vi "Periodic Tasks.vi"(8 "error in":errorcluster) -> ()   [LabVIEW 2015]
doc: "This VI runs in parallel to other tasks. It can contain as many user-defined periodic loops as you need. These can carry out PID or other sorts of timed response."
uses:
  Robot Global Data.vi
  <vilib>/Rock Robotics/WPI/Ultrasonic/WPI_SonarMB1010DigitalRefNum Registry Get.vi
  <vilib>/Rock Robotics/WPI/Ultrasonic/WPI_SonarMB1010DigitalGetRange.vi
  <vilib>/addons/control/pid/pid.llb/PID (DBL).vi
  navx-mxp/labview/navX Library v2/navX Library v2.lvlib
  <vilib>/addons/control/pid/NI_PID_pid.lvlib
panel:
  in  "Amperage setpoint":dbl=4.5 format="%#_13g"
  out "current (A)":dbl
  out "Pitch":dbl
  in  "PID gains 2":T1={"proportional gain (Kc)"=6.0, "integral time (Ti, min)"=0.0, "derivative time (Td, min)"=0.0}
  in  "Level 1":dbl=0.106 format="%#_13g"
  in  "Level 2":dbl=0.2 format="%#_13g"
  in  "Level 3":dbl=0.845 format="%#_13g"
  out "Motor Output":dbl(graph)
  in  "PID gains":T1={"proportional gain (Kc)"=7.0, "integral time (Ti, min)"=0.0, "derivative time (Td, min)"=0.00045}
  out "Distance":dbl
  out "Potentiometer":dbl
  out "Beam Brake Tripped?":bool
  out "Yaw":dbl
  out "Roll":dbl
  in  "Command limit":dbl=0.25
  in  "Yaw Reset":bool
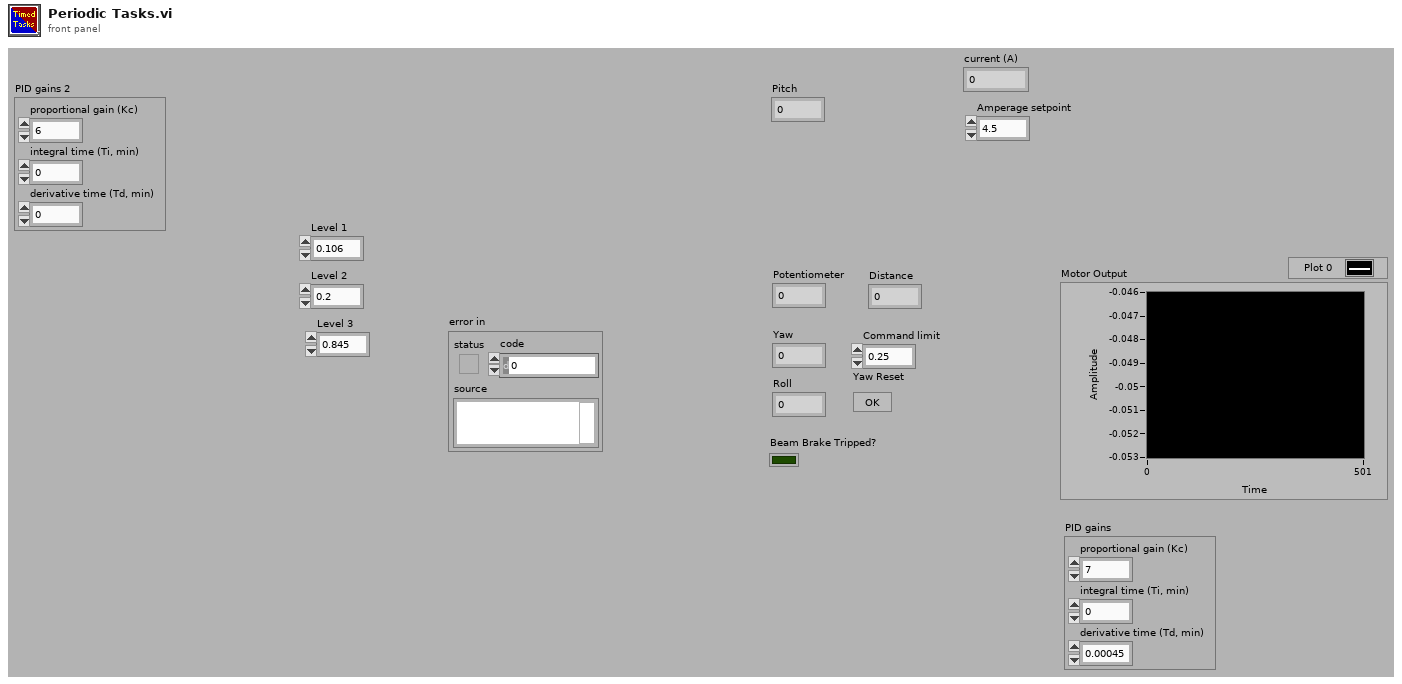
[diagram p1: front panel]
types:
  T1 = cluster{"proportional gain (Kc)":dbl, "integral time (Ti, min)":dbl, "derivative time (Td, min)":dbl}
  T2 = typedef "WPI_MotorControlDeviceRef.ctl" = cluster{"DeviceStatus":errorcluster, "Type":T3, "PWM":cluster{"PWM Channel":T4, "DeadBand":T5}, "CAN":cluster{"Device Number":u8, "Control Mode":T6, "Semaphore":T7, "Max Vout":dbl, "TalonSRX Control Mode":T8}, "Invert":bool}
  T3 = typedef "WPI_MotorControlType.ctl" = enum16{"PWM", "CAN", "CANTalonSRX"}
  T4 = typedef "FPGA_DIOPWMChannel.ctl" = enum8{"PWM 0", "PWM 1", "PWM 2", "PWM 3", "PWM 4", "PWM 5", "PWM 6", "PWM 7", "PWM 8", "PWM 9", "PWM MXP 0", "PWM MXP 1", "PWM MXP 2", "PWM MXP 3", "PWM MXP 4", "PWM MXP 5", "PWM MXP 6", "PWM MXP 7", "PWM MXP 8", "PWM MXP 9", "Invalid"}
  T5 = typedef "WPI_PWMDeadband.ctl" = cluster{"Name":string, "maxPositivePwm":i32, "minPositivePwm":i32, "centerPwm":i32, "maxNegativePwm":i32, "minNegativePwm":i32, "angularRange":u16}
  T6 = typedef "WPI_CANJaguar_ControlMode.ctl" = enum8{"Percent VBus", "Current", "Speed", "Position", "Voltage"}
  T7 = typedef "Semaphore RefNum" = refnum<k1>
  T8 = typedef "WPI_CANTalonSRX_APIControlMode.ctl" = enum8{"Percent VBus", "Speed", "Position", "Slave", "Unchanged / Invalid", "Voltage Compensation", "Current", "Motion Profile"}
  T9 = typedef "WPI_PotentiometerDevRef.ctl" = cluster{"DevStatus":errorcluster, "Analog Channel":T10, "Invert Output":bool}
  T10 = typedef "FPGA_AIChannel.ctl" = enum8{"AI 0", "AI 1", "AI 2", "AI 3", "AI MXP 0", "AI MXP 1", "AI MXP 2", "AI MXP 3", "Invalid"}
  T11 = typedef "WPI_DigitalInputDevRef.ctl" = cluster{"DevStatus":errorcluster, "DIO Channel":T12}
  T12 = typedef "FPGA_DIOChannel.ctl" = enum8{"DIO 0", "DIO 1", "DIO 2", "DIO 3", "DIO 4", "DIO 5", "DIO 6", "DIO 7", "DIO 8", "DIO 9", "DIO MXP 0", "DIO MXP 1", "DIO MXP 2", "DIO MXP 3", "DIO MXP 4", "DIO MXP 5", "DIO MXP 6", "DIO MXP 7", "DIO MXP 8", "DIO MXP 9", "DIO MXP 10", "DIO MXP 11", "DIO MXP 12", "DIO MXP 13", "DIO MXP 14", "DIO MXP 15", "Invalid"}
  T13 = typedef "WPI_SonarMB1010DigitalDeviceRef.ctl" = cluster{"CounterDevRef":T14, "Scaling factor (s/in)":dbl}
  T14 = typedef "WPI_CounterDevRef.ctl" = cluster{"DevStatus":errorcluster, "CntIndex":T15}
  T15 = typedef "FPGA_CounterCtrSystemIndex.ctl" = enum8{"Ctr 0", "Ctr 1", "Ctr 2", "Ctr 3", "Ctr 4", "Ctr 5", "Ctr 6", "Ctr 7", "Invalid"}
  T16 = typedef "navX Library v2.lvlib/Z900_navX_DeviceTypeDef.ctl" = cluster{"Interface":cluster{"Protocol":T17, "Update Rate (4Hz-60Hz)":u8, "navX Open TypeDef":variant}, "Notify Packet":refnum<notifier>, "Loop VI Refnum":refnum<vi>, "Ready to Close Occurrence Refnum":refnum<k4>}
  T17 = typedef "navX Library v2.lvlib/Z900_navX_ProtocolTypeDef.ctl" = enum16{"SERIAL", "I2C", "SPI"}
  T18 = cluster{"Yaw":dbl, "Roll":dbl, "Pitch":dbl, "Heading":dbl, "Fused Heading":dbl}
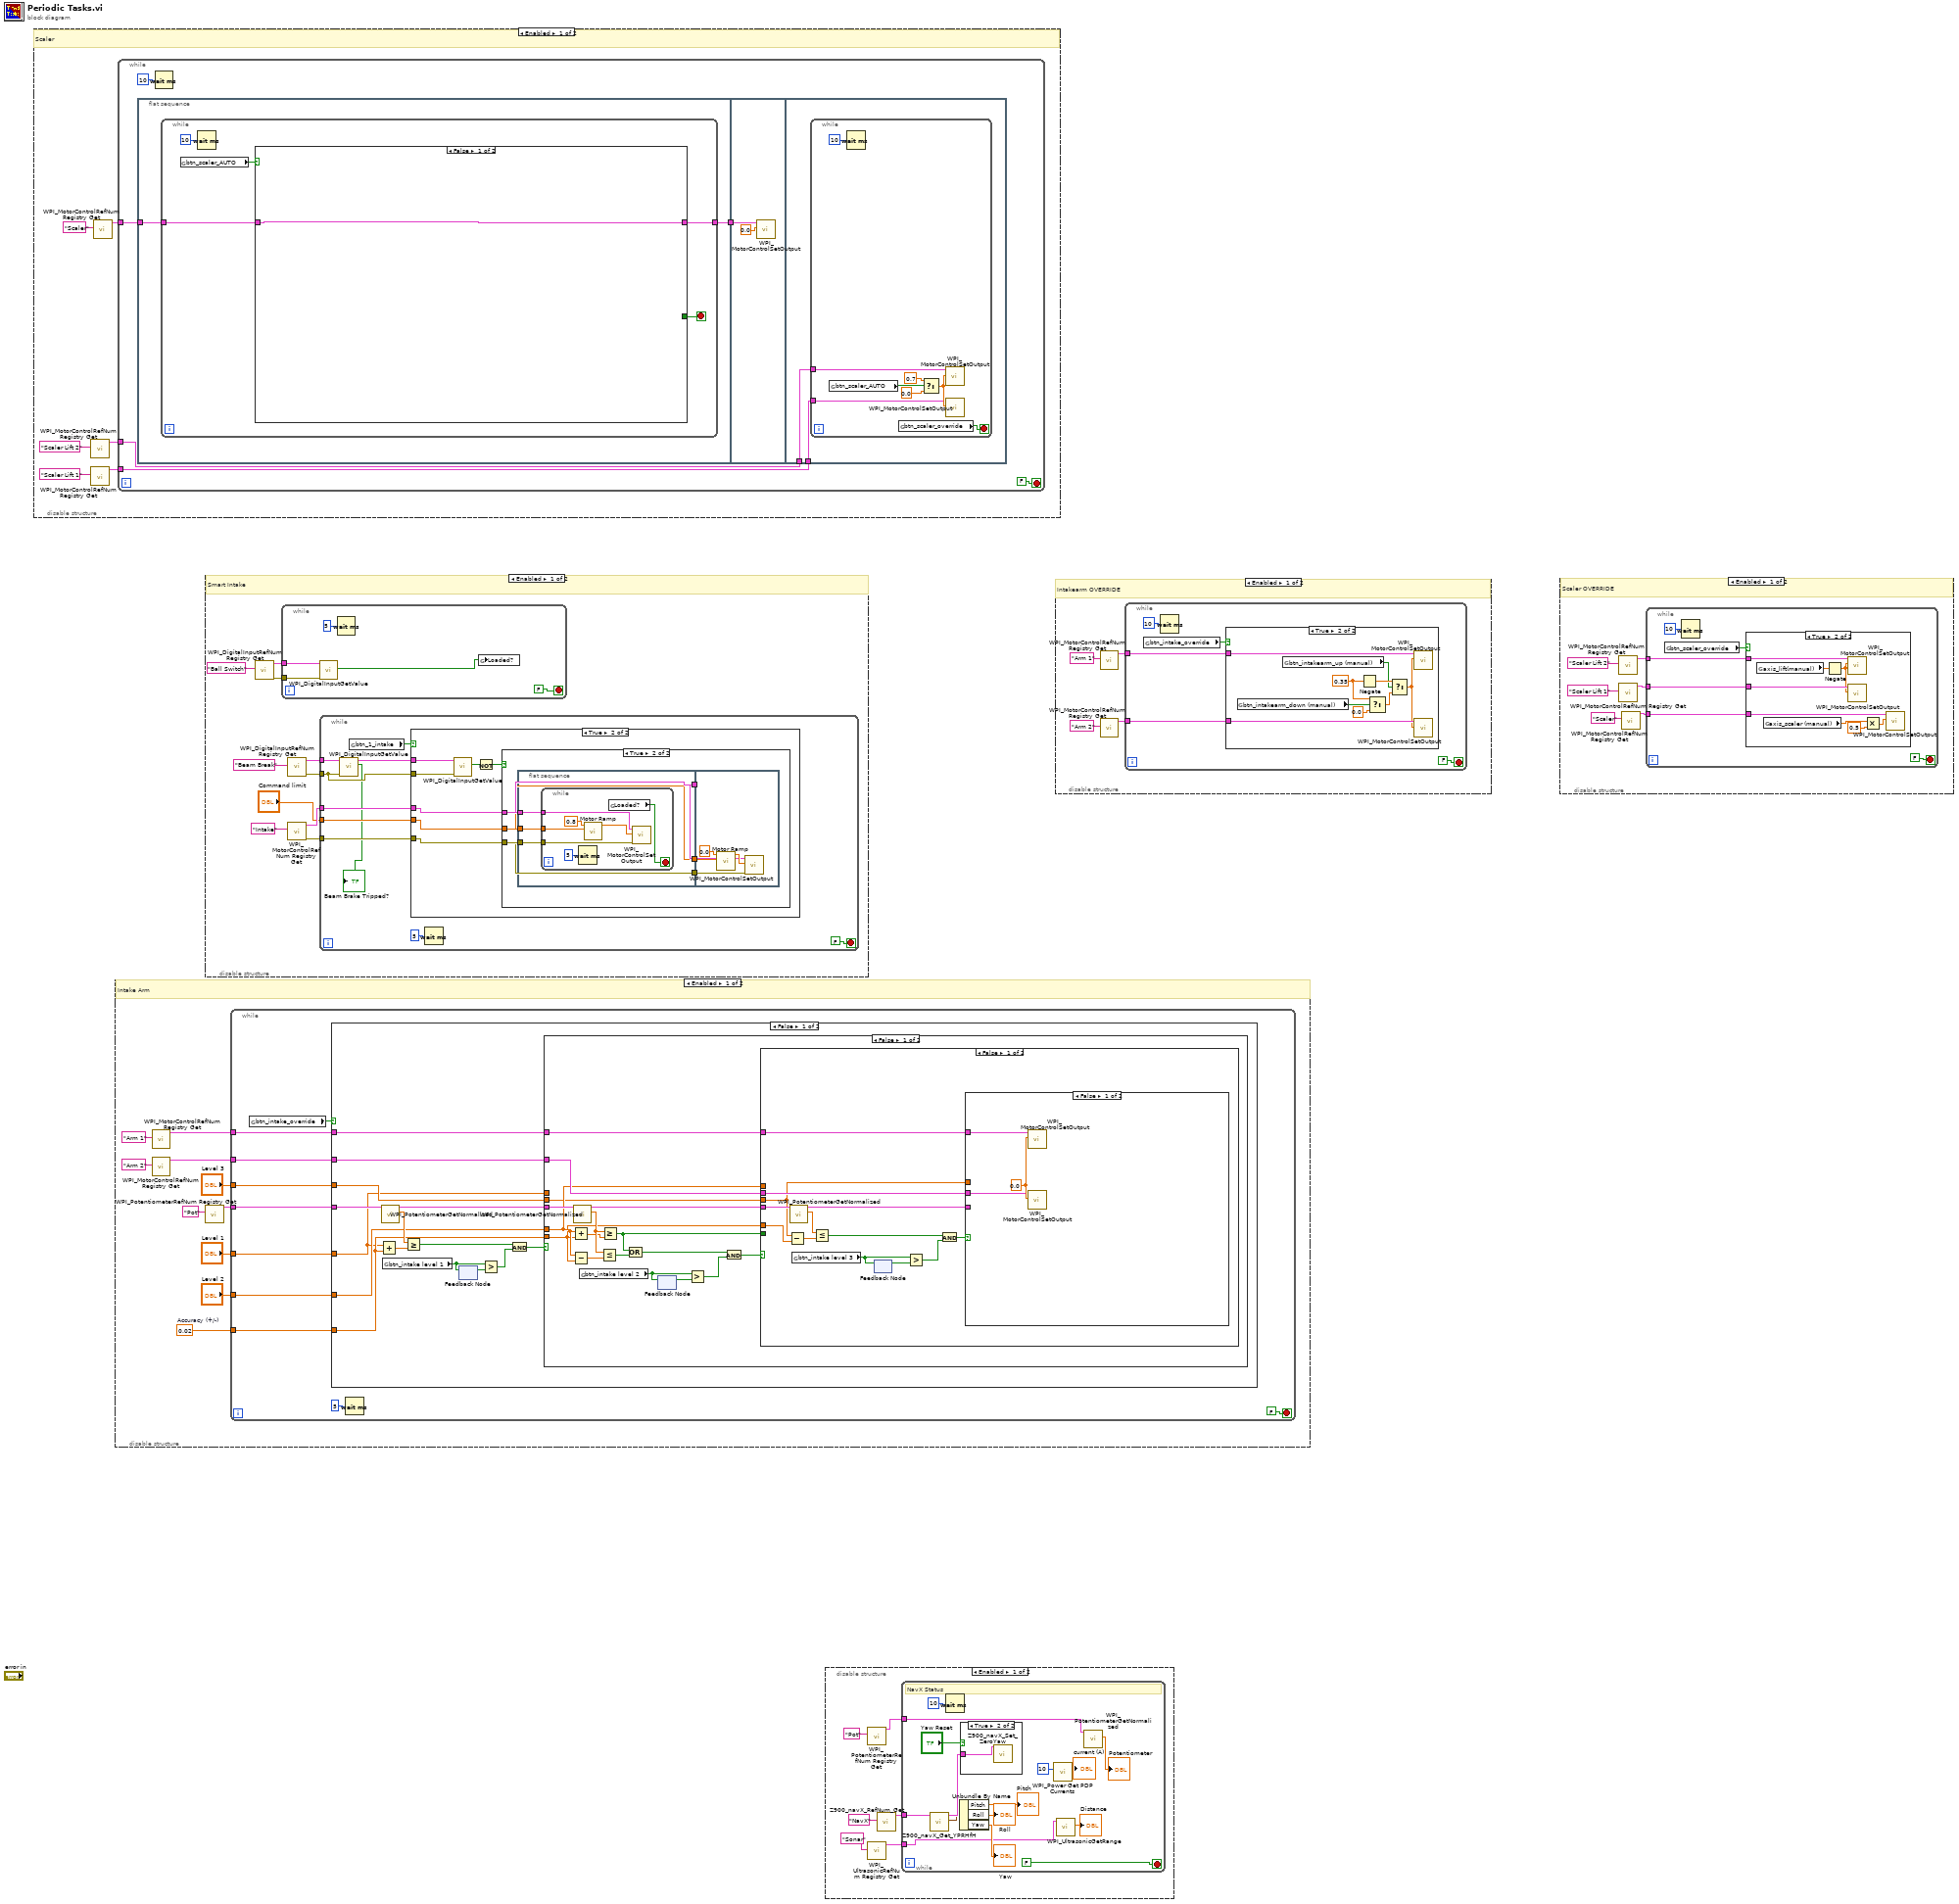
[diagram p0: block diagram]
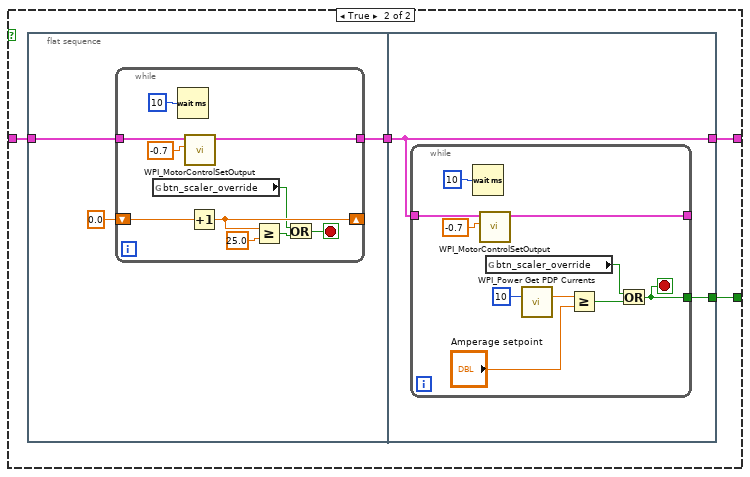
[diagram p2: hidden frame]
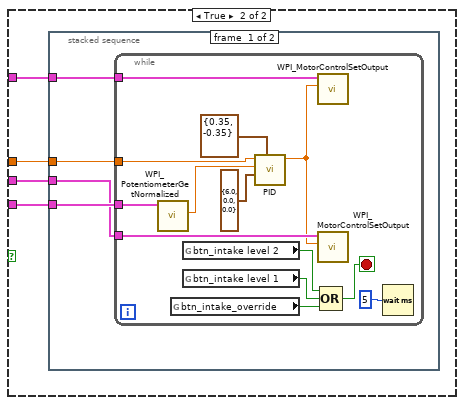
[diagram p8: hidden frame]
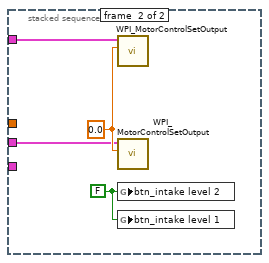
[diagram p9: hidden frame]
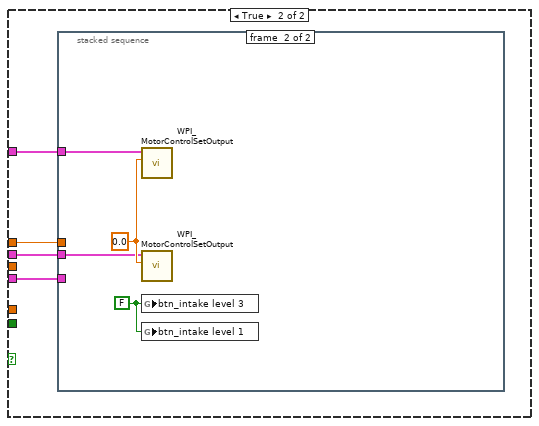
[diagram p10: hidden frame]
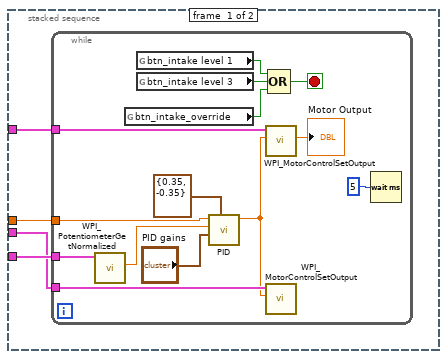
[diagram p11: hidden frame]
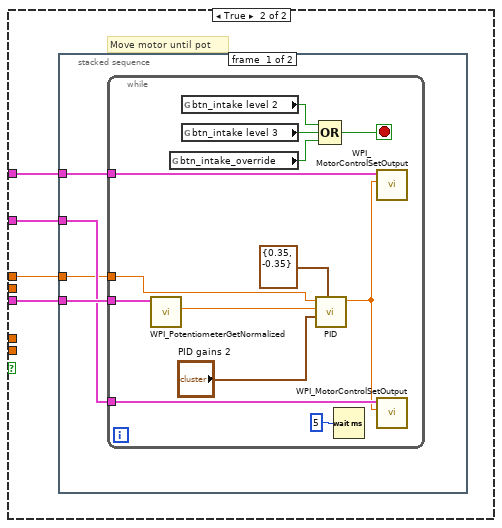
[diagram p12: hidden frame]
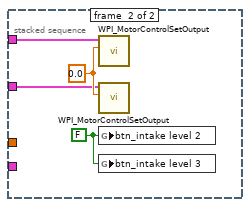
[diagram p13: hidden frame]
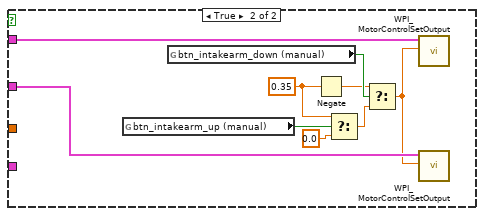
[diagram p14: hidden frame]
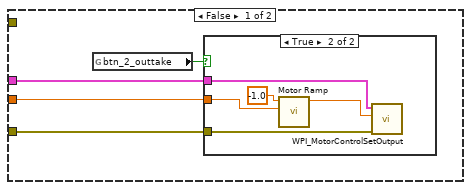
[diagram p18: hidden frame]
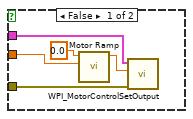
[diagram p19: hidden frame]
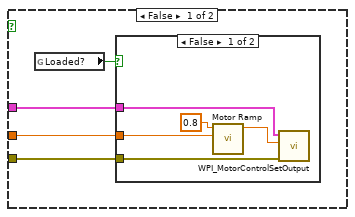
[diagram p20: hidden frame]
diagram:
  n1 = disable-structure shown="Enabled" {
    frame Enabled {
      # "Scaler"
      n2 = call <vilib>:"WPI_MotorControlRefNum Registry Get.vi"("refnum name"="Scaler Lift 2") -> ("MotorControlDevRef"=w2:T2)  [unwired: 9 in, 1 out]
      n3 = call <vilib>:"WPI_MotorControlRefNum Registry Get.vi"("refnum name"="Scaler Lift 1") -> ("MotorControlDevRef"=w1:T2)  [unwired: 9 in, 1 out]
      n4 = call <vilib>:"WPI_MotorControlRefNum Registry Get.vi"("refnum name"="Scaler") -> ("MotorControlDevRef"=w3:T2)  [unwired: 9 in, 1 out]
      n5 = while {
        tunnel: w3 -> [w10]
        tunnel: w2 -> [w8]
        tunnel: w1 -> [w7]
        stop <- FALSE stop-if-true
        n6 = flat-sequence {
          tunnel: w10 -> [w14]
          tunnel: [w13] -> w9
          tunnel: w9 -> [w51]
          tunnel: w8 -> [w53]
          tunnel: w7 -> [w52]
          frame #0 {
            n7 = while {
              tunnel: w14 -> [w18]
              tunnel: [w17] -> w13
              stop <- w16 stop-if-true
              n8 = global read "Robot Global Data.vi" "btn_scaler_AUTO"() -> (w19:bool)
              n9 = Wait (ms)(milliseconds to wait=u32 10) -> ()  [unwired: 1 out]
              n10 = case shown="False" w19 {
                tunnel: w18 -> [w20 w24]
                tunnel: [w20 w23] -> w17
                tunnel: [_ w21] -> w16
                frame False {
                }
                frame True {
                  n11 = flat-sequence {
                    tunnel: w24 -> [w27]
                    tunnel: [w26] -> w22
                    tunnel: [w39] -> w23
                    tunnel: w22 -> [w39]
                    tunnel: [w38] -> w21
                    frame #0 {
                      n12 = while {
                        tunnel: w27 -> [w37]
                        tunnel: [w36] -> w26
                        shift-right: [w31] -> _
                        shift-left: 0.0 -> [w33]
                        stop <- w30 stop-if-true
                        n13 = global read "Robot Global Data.vi" "btn_scaler_override"() -> (w29:bool)
                        n14 = Wait (ms)(milliseconds to wait=u32 10) -> ()  [unwired: 1 out]
                        n15 = call <vilib>:"WPI_MotorControlSetOutput.vi"("Output"=-0.7, "MotorControlDevRef"=w37) -> ("MotorControlDevRef"=w36:T2)  [unwired: 7 in, 2 out]
                        n16 = Increment(x=w33) -> (x+1=w31:dbl)
                        n17 = Greater Or Equal?(x=w31, y=25.0) -> (x >= y?=w28:bool)
                        n18 = Or(x=w29, y=w28) -> (x .or. y?=w30:bool)
                      }
                    }
                    frame #1 {
                      n19 = while {
                        tunnel: [w49] -> _
                        tunnel: w39 -> [w45]
                        tunnel: [w40] -> w38
                        stop <- w40 stop-if-true
                        n20 = Wait (ms)(milliseconds to wait=u32 10) -> ()  [unwired: 1 out]
                        n21 = call <vilib>:"WPI_MotorControlSetOutput.vi"("Output"=-0.7, "MotorControlDevRef"=w45) -> ("MotorControlDevRef"=w49:T2)  [unwired: 7 in, 2 out]
                        n22 = global read "Robot Global Data.vi" "btn_scaler_override"() -> (w46:bool)
                        n23 = call <vilib>:"WPI_Power Get PDP Currents.vi"("PDP Channel"=10) -> ("current (A)"=w43:dbl)  [unwired: 12 in, 2 out]
                        n24 = Greater Or Equal?(x=w43, y="Amperage setpoint") -> (x >= y?=w42:bool)
                        n25 = Or(x=w46, y=w42) -> (x .or. y?=w40:bool)
                      }
                    }
                  }
                }
              }
            }
          }
          frame #1 {
            n26 = call <vilib>:"WPI_MotorControlSetOutput.vi"("Output"=0.0, "MotorControlDevRef"=w51) -> ()  [unwired: 7 in, 3 out]
          }
          frame #2 {
            n27 = while {
              tunnel: w53 -> [w55]
              tunnel: w52 -> [w54]
              stop <- w60 stop-if-true
              n28 = global read "Robot Global Data.vi" "btn_scaler_AUTO"() -> (w59:bool)
              n29 = Wait (ms)(milliseconds to wait=u32 10) -> ()  [unwired: 1 out]
              n30 = global read "Robot Global Data.vi" "btn_scaler_override"() -> (w60:bool)
              n31 = Select(t=0.7, s=w59, f=0.0) -> (s? t:f=w56:dbl)
              n32 = call <vilib>:"WPI_MotorControlSetOutput.vi"("Output"=w56, "MotorControlDevRef"=w55) -> ()  [unwired: 7 in, 3 out]
              n33 = call <vilib>:"WPI_MotorControlSetOutput.vi"("Output"=w56, "MotorControlDevRef"=w54) -> ()  [unwired: 7 in, 3 out]
            }
          }
        }
        n34 = Wait (ms)(milliseconds to wait=u32 10) -> ()  [unwired: 1 out]
      }
    }
    frame Disabled {
    }
  }
  n35 = disable-structure shown="Enabled" {
    frame Enabled {
      w65 = 0.02  # Accuracy (+/-)
      # "Intake Arm"
      n36 = call <vilib>:"WPI_MotorControlRefNum Registry Get.vi"("refnum name"="Arm 1") -> ("MotorControlDevRef"=w67:T2)  [unwired: 9 in, 1 out]
      n37 = call <vilib>:"WPI_MotorControlRefNum Registry Get.vi"("refnum name"="Arm 2") -> ("MotorControlDevRef"=w66:T2)  [unwired: 9 in, 1 out]
      n38 = call <vilib>:"WPI_PotentiometerRefNum Registry Get.vi"("refnum name"="Pot") -> ("PotDevRef"=w68:T9)  [unwired: 9 in, 1 out]
      n39 = while {
        tunnel: w68 -> [w80]
        tunnel: w67 -> [w79]
        tunnel: w66 -> [w78]
        tunnel: w65 -> [w76]
        tunnel: "Level 3" -> [w75]
        tunnel: "Level 2" -> [w74]
        tunnel: "Level 1" -> [w73]
        stop <- FALSE stop-if-true
        n40 = global read "Robot Global Data.vi" "btn_intake_override"() -> (w72:bool)
        n41 = case shown="False" w72 {
          tunnel: w80 -> [w91 _]
          tunnel: w79 -> [w89 w214]
          tunnel: w78 -> [w88 w213]
          tunnel: w76 -> [w85 _]
          tunnel: w75 -> [w84 _]
          tunnel: w74 -> [w83 _]
          tunnel: w73 -> [w82 _]
          frame False {
            n42 = Add(x=w82, y=w85) -> (x+y=w86:dbl)
            n43 = call <vilib>:"WPI_PotentiometerGetNormalized.vi"("PotDevRef"=w91) -> ("Normalized Value"=w87:dbl, "PotDevRef"=w90:T9)  [unwired: 8 in, 1 out]
            n44 = global read "Robot Global Data.vi" "btn_intake level 1"() -> (w92:bool)
            n45 = Greater Or Equal?(x=w87, y=w86) -> (x >= y?=w95:bool)
            n46 = feedback #1() -> (w93:bool)  [unwired: 1 in]
            n47 = feedback-in #1(w92) -> ()
            n48 = Greater?(x=w92, y=w93) -> (0:w94:bool)
            n49 = And(x=w95, y=w94) -> (x .and. y?=w96:bool)
            n50 = case shown="False" w96 {
              tunnel: w90 -> [w106 w184]
              tunnel: w89 -> [w103 w183]
              tunnel: w88 -> [w102 w182]
              tunnel: w83 -> [w99 _]
              tunnel: w85 -> [w98 _]
              tunnel: w84 -> [w97 _]
              tunnel: w82 -> [_ w181]
              frame False {
                n51 = Add(x=w99, y=w98) -> (x+y=w101:dbl)
                n52 = Subtract(x=w99, y=w98) -> (x-y=w100:dbl)
                n53 = call <vilib>:"WPI_PotentiometerGetNormalized.vi"("PotDevRef"=w106) -> ("Normalized Value"=w107:dbl, "PotDevRef"=w105:T9)  [unwired: 8 in, 1 out]
                n54 = global read "Robot Global Data.vi" "btn_intake level 2"() -> (w108:bool)
                n55 = Less Or Equal?(x=w107, y=w100) -> (x <= y?=w112:bool)
                n56 = Greater Or Equal?(x=w107, y=w101) -> (x >= y?=w104:bool)
                n57 = Or(x=w104, y=w112) -> (x .or. y?=w110:bool)
                n58 = feedback #2() -> (w113:bool)  [unwired: 1 in]
                n59 = feedback-in #2(w108) -> ()
                n60 = Greater?(x=w108, y=w113) -> (0:w111:bool)
                n61 = And(x=w110, y=w111) -> (x .and. y?=w109:bool)
                n62 = case shown="False" w109 {
                  tunnel: w105 -> [w120 w158]
                  tunnel: w104 -> [_ _]
                  tunnel: w103 -> [w117 w157]
                  tunnel: w102 -> [w118 w156]
                  tunnel: w99 -> [_ w155]
                  tunnel: w98 -> [w115 _]
                  tunnel: w97 -> [w114 _]
                  frame False {
                    n63 = Subtract(x=w114, y=w115) -> (x-y=w116:dbl)
                    n64 = call <vilib>:"WPI_PotentiometerGetNormalized.vi"("PotDevRef"=w120) -> ("Normalized Value"=w121:dbl, "PotDevRef"=w119:T9)  [unwired: 8 in, 1 out]
                    n65 = global read "Robot Global Data.vi" "btn_intake level 3"() -> (w122:bool)
                    n66 = Less Or Equal?(x=w121, y=w116) -> (x <= y?=w124:bool)
                    n67 = feedback #3() -> (w126:bool)  [unwired: 1 in]
                    n68 = feedback-in #3(w122) -> ()
                    n69 = Greater?(x=w122, y=w126) -> (0:w125:bool)
                    n70 = And(x=w124, y=w125) -> (x .and. y?=w123:bool)
                    n71 = case shown="False" w123 {
                      tunnel: w119 -> [_ w133]
                      tunnel: w118 -> [w127 w132]
                      tunnel: w117 -> [w128 w131]
                      tunnel: w114 -> [_ w130]
                      frame False {
                        w129 = 0.0 ("Output")
                        n72 = call <vilib>:"WPI_MotorControlSetOutput.vi"("Output"=w129, "MotorControlDevRef"=w128) -> ()  [unwired: 7 in, 3 out]
                        n73 = call <vilib>:"WPI_MotorControlSetOutput.vi"("Output"=w129, "MotorControlDevRef"=w127) -> ()  [unwired: 7 in, 3 out]
                      }
                      frame True {
                        n74 = stacked-sequence {
                          tunnel: w133 -> [w137 _]
                          tunnel: w132 -> [w136 w153]
                          tunnel: w131 -> [w135 w152]
                          tunnel: w130 -> [w134 _]
                          frame #0 {
                            n75 = while {
                              tunnel: w137 -> [w149]
                              tunnel: w136 -> [w148]
                              tunnel: w135 -> [w147]
                              tunnel: w134 -> [w139]
                              stop <- w140 stop-if-true
                              n76 = call <vilib>:"WPI_PotentiometerGetNormalized.vi"("PotDevRef"=w149) -> ("Normalized Value"=w143:dbl)  [unwired: 8 in, 2 out]
                              n77 = global read "Robot Global Data.vi" "btn_intake_override"() -> (w138:bool)
                              n78 = global read "Robot Global Data.vi" "btn_intake level 2"() -> (w142:bool)
                              n79 = global read "Robot Global Data.vi" "btn_intake level 1"() -> (w141:bool)
                              n80 = call-poly <vilib>:"PID.vi"("output range"=cluster{"output high":dbl, "output low":dbl} {"output high"=0.35, "output low"=-0.35}, "PID gains"=T1 {"proportional gain (Kc)"=6.0, "integral time (Ti, min)"=0.0, "derivative time (Td, min)"=0.0}, "process variable"=w143, "setpoint"=w139) -> ("output"=w146:dbl)  [unwired: 6 in, 1 out]
                              n81 = call <vilib>:"WPI_MotorControlSetOutput.vi"("Output"=w146, "MotorControlDevRef"=w147) -> ()  [unwired: 7 in, 3 out]
                              n82 = call <vilib>:"WPI_MotorControlSetOutput.vi"("Output"=w146, "MotorControlDevRef"=w148) -> ()  [unwired: 7 in, 3 out]
                              n83 = Compound Arithmetic op=OR(w142, w141, w138) -> (w140:bool)
                              n84 = Wait (ms)(milliseconds to wait=u32 5) -> ()  [unwired: 1 out]
                            }
                          }
                          frame #1 {
                            w151 = FALSE ("btn_intake level 2")
                            w154 = 0.0 ("Output")
                            n85 = call <vilib>:"WPI_MotorControlSetOutput.vi"("Output"=w154, "MotorControlDevRef"=w152) -> ()  [unwired: 7 in, 3 out]
                            n86 = call <vilib>:"WPI_MotorControlSetOutput.vi"("Output"=w154, "MotorControlDevRef"=w153) -> ()  [unwired: 7 in, 3 out]
                            n87 = global write "Robot Global Data.vi" "btn_intake level 2"(w151) -> ()
                            n88 = global write "Robot Global Data.vi" "btn_intake level 1"(w151) -> ()
                          }
                        }
                      }
                    }
                  }
                  frame True {
                    n89 = stacked-sequence {
                      tunnel: w158 -> [w162 _]
                      tunnel: w157 -> [w161 w178]
                      tunnel: w156 -> [w160 w179]
                      tunnel: w155 -> [w159 _]
                      frame #0 {
                        n90 = while {
                          tunnel: w162 -> [w175]
                          tunnel: w161 -> [w174]
                          tunnel: w160 -> [w173]
                          tunnel: w159 -> [w165]
                          stop <- w166 stop-if-true
                          n91 = call <vilib>:"WPI_PotentiometerGetNormalized.vi"("PotDevRef"=w175) -> ("Normalized Value"=w169:dbl)  [unwired: 8 in, 2 out]
                          n92 = global read "Robot Global Data.vi" "btn_intake_override"() -> (w163:bool)
                          n93 = global read "Robot Global Data.vi" "btn_intake level 1"() -> (w168:bool)
                          n94 = global read "Robot Global Data.vi" "btn_intake level 3"() -> (w167:bool)
                          n95 = call-poly <vilib>:"PID.vi"("output range"=cluster{"output high":dbl, "output low":dbl} {"output high"=0.35, "output low"=-0.35}, "PID gains"="PID gains", "process variable"=w169, "setpoint"=w165) -> ("output"=w170:dbl)  [unwired: 6 in, 1 out]
                          n96 = call <vilib>:"WPI_MotorControlSetOutput.vi"("Output"=w170, "MotorControlDevRef"=w174) -> ("Motor Output"=→"Motor Output":dbl)  [unwired: 7 in, 2 out]
                          n97 = call <vilib>:"WPI_MotorControlSetOutput.vi"("Output"=w170, "MotorControlDevRef"=w173) -> ()  [unwired: 7 in, 3 out]
                          n98 = Compound Arithmetic op=OR(w168, w167, w163) -> (w166:bool)
                          n99 = Wait (ms)(milliseconds to wait=u32 5) -> ()  [unwired: 1 out]
                        }
                      }
                      frame #1 {
                        w177 = FALSE ("btn_intake level 2")
                        w180 = 0.0 ("Output")
                        n100 = call <vilib>:"WPI_MotorControlSetOutput.vi"("Output"=w180, "MotorControlDevRef"=w178) -> ()  [unwired: 7 in, 3 out]
                        n101 = call <vilib>:"WPI_MotorControlSetOutput.vi"("Output"=w180, "MotorControlDevRef"=w179) -> ()  [unwired: 7 in, 3 out]
                        n102 = global write "Robot Global Data.vi" "btn_intake level 3"(w177) -> ()
                        n103 = global write "Robot Global Data.vi" "btn_intake level 1"(w177) -> ()
                      }
                    }
                  }
                }
              }
              frame True {
                # "Move motor until pot"
                n104 = stacked-sequence {
                  tunnel: w184 -> [w188 _]
                  tunnel: w183 -> [w187 w204]
                  tunnel: w182 -> [w186 w203]
                  tunnel: w181 -> [w185 _]
                  frame #0 {
                    n105 = while {
                      tunnel: w188 -> [w200]
                      tunnel: w187 -> [w199]
                      tunnel: w186 -> [w198]
                      tunnel: w185 -> [w190]
                      stop <- w191 stop-if-true
                      n106 = call <vilib>:"WPI_PotentiometerGetNormalized.vi"("PotDevRef"=w200) -> ("Normalized Value"=w192:dbl)  [unwired: 8 in, 2 out]
                      n107 = global read "Robot Global Data.vi" "btn_intake_override"() -> (w189:bool)
                      n108 = global read "Robot Global Data.vi" "btn_intake level 2"() -> (w195:bool)
                      n109 = global read "Robot Global Data.vi" "btn_intake level 3"() -> (w194:bool)
                      n110 = call-poly <vilib>:"PID.vi"("output range"=cluster{"output high":dbl, "output low":dbl} {"output high"=0.35, "output low"=-0.35}, "PID gains"="PID gains 2", "process variable"=w192, "setpoint"=w190) -> ("output"=w193:dbl)  [unwired: 6 in, 1 out]
                      n111 = Compound Arithmetic op=OR(w195, w194, w189) -> (w191:bool)
                      n112 = Wait (ms)(milliseconds to wait=u32 5) -> ()  [unwired: 1 out]
                      n113 = call <vilib>:"WPI_MotorControlSetOutput.vi"("Output"=w193, "MotorControlDevRef"=w199) -> ()  [unwired: 7 in, 3 out]
                      n114 = call <vilib>:"WPI_MotorControlSetOutput.vi"("Output"=w193, "MotorControlDevRef"=w198) -> ()  [unwired: 7 in, 3 out]
                    }
                  }
                  frame #1 {
                    w202 = FALSE ("btn_intake level 2")
                    w205 = 0.0 ("Output")
                    n115 = call <vilib>:"WPI_MotorControlSetOutput.vi"("Output"=w205, "MotorControlDevRef"=w204) -> ()  [unwired: 7 in, 3 out]
                    n116 = call <vilib>:"WPI_MotorControlSetOutput.vi"("Output"=w205, "MotorControlDevRef"=w203) -> ()  [unwired: 7 in, 3 out]
                    n117 = global write "Robot Global Data.vi" "btn_intake level 2"(w202) -> ()
                    n118 = global write "Robot Global Data.vi" "btn_intake level 3"(w202) -> ()
                  }
                }
              }
            }
          }
          frame True {
            w207 = 0.35 ("t")
            n119 = global read "Robot Global Data.vi" "btn_intakearm_up (manual)"() -> (w210:bool)
            n120 = global read "Robot Global Data.vi" "btn_intakearm_down (manual)"() -> (w209:bool)
            n121 = Negate(x=w207) -> (-x=w206:dbl)
            n122 = Select(t=w207, s=w210, f=0.0) -> (s? t:f=w212:dbl)
            n123 = Select(t=w206, s=w209, f=w212) -> (s? t:f=w211:dbl)
            n124 = call <vilib>:"WPI_MotorControlSetOutput.vi"("Output"=w211, "MotorControlDevRef"=w214) -> ()  [unwired: 7 in, 3 out]
            n125 = call <vilib>:"WPI_MotorControlSetOutput.vi"("Output"=w211, "MotorControlDevRef"=w213) -> ()  [unwired: 7 in, 3 out]
          }
        }
        n126 = Wait (ms)(milliseconds to wait=u32 5) -> ()  [unwired: 1 out]
      }
    }
    frame Disabled {
    }
  }
  n127 = disable-structure shown="Enabled" {
    frame Enabled {
      # "Smart Intake"
      n128 = call <vilib>:"WPI_DigitalInputRefNum Registry Get.vi"("refnum name"="Ball Switch") -> ("error out"=w216:errorcluster, "DigitalInputDevRef"=w215:T11)  [unwired: 9 in]
      n129 = while {
        tunnel: w216 -> [w229]
        tunnel: w215 -> [w228]
        stop <- FALSE stop-if-true
        n130 = call <vilib>:"WPI_DigitalInputGetValue.vi"("error in (no error)"=w229, "DigitalInputDevRef"=w228) -> ("Value"=w225:bool)  [unwired: 7 in, 2 out]
        n131 = Wait (ms)(milliseconds to wait=u32 5) -> ()  [unwired: 1 out]
        n132 = global write "Robot Global Data.vi" "Loaded?"(w225) -> ()
      }
      n133 = call <vilib>:"WPI_DigitalInputRefNum Registry Get.vi"("refnum name"="Beam Break") -> ("error out"=w224:errorcluster, "DigitalInputDevRef"=w223:T11)  [unwired: 9 in]
      n134 = call <vilib>:"WPI_MotorControlRefNum Registry Get.vi"("refnum name"="Intake") -> ("error out"=w221:errorcluster, "MotorControlDevRef"=w220:T2)  [unwired: 9 in]
      n135 = while {
        tunnel: w223 -> [w239]
        tunnel: w224 -> [w231]
        tunnel: w220 -> [w238]
        tunnel: w221 -> [w237]
        tunnel: "Command limit" -> [w236]
        stop <- FALSE stop-if-true
        n136 = call <vilib>:"WPI_DigitalInputGetValue.vi"("error in (no error)"=w231, "DigitalInputDevRef"=w239) -> ("Value"=→"Beam Brake Tripped?":bool, "DigitalInputDevRef"=w232:T11)  [unwired: 7 in, 1 out]
        n137 = global read "Robot Global Data.vi" "btn_1_intake"() -> (w235:bool)
        n138 = case shown="True" w235 {
          tunnel: w232 -> [_ w260]
          tunnel: w231 -> [_ w259]
          tunnel: w238 -> [w243 w258]
          tunnel: w237 -> [w242 w257]
          tunnel: w236 -> [w241 w256]
          frame False {
            n139 = global read "Robot Global Data.vi" "btn_2_outtake"() -> (w240:bool)
            n140 = case shown="True" w240 {
              tunnel: w241 -> [w248 w253]
              tunnel: w243 -> [w247 w252]
              tunnel: w242 -> [w246 w251]
              frame False {
                n141 = call "Motor Ramp.vi"("Command limit"=w248, "Joystick in"=0.0) -> ("Joystick out"=w245:dbl)  [unwired: 9 in]
                n142 = call <vilib>:"WPI_MotorControlSetOutput.vi"("error in (no error)"=w246, "Output"=w245, "MotorControlDevRef"=w247) -> ()  [unwired: 6 in, 3 out]
              }
              frame True {
                n143 = call "Motor Ramp.vi"("Command limit"=w253, "Joystick in"=-1.0) -> ("Joystick out"=w250:dbl)  [unwired: 9 in]
                n144 = call <vilib>:"WPI_MotorControlSetOutput.vi"("error in (no error)"=w251, "Output"=w250, "MotorControlDevRef"=w252) -> ()  [unwired: 6 in, 3 out]
              }
            }
          }
          frame True {
            n145 = call <vilib>:"WPI_DigitalInputGetValue.vi"("error in (no error)"=w259, "DigitalInputDevRef"=w260) -> ("Value"=w254:bool)  [unwired: 7 in, 2 out]
            n146 = Not(x=w254) -> (.not. x?=w255:bool)
            n147 = case shown="True" w255 {
              tunnel: w258 -> [w264 w272]
              tunnel: w257 -> [w263 w271]
              tunnel: w256 -> [w262 w270]
              frame False {
                n148 = global read "Robot Global Data.vi" "Loaded?"() -> (w261:bool)
                n149 = case shown="False" w261 {
                  tunnel: w262 -> [w267 _]
                  tunnel: w264 -> [w269 _]
                  tunnel: w263 -> [w265 _]
                  frame False {
                    n150 = call "Motor Ramp.vi"("Command limit"=w267, "Joystick in"=0.8 ("Command limit")) -> ("Joystick out"=w268:dbl)  [unwired: 9 in]
                    n151 = call <vilib>:"WPI_MotorControlSetOutput.vi"("error in (no error)"=w265, "Output"=w268, "MotorControlDevRef"=w269) -> ()  [unwired: 6 in, 3 out]
                  }
                  frame True {
                  }
                }
              }
              frame True {
                n152 = flat-sequence {
                  tunnel: w272 -> [w278]
                  tunnel: w271 -> [w277]
                  tunnel: w270 -> [w276]
                  tunnel: [w278] -> w275
                  tunnel: [w277] -> w274
                  tunnel: [w276] -> w273
                  tunnel: w275 -> [w286]
                  tunnel: w274 -> [w290]
                  tunnel: w273 -> [w289]
                  frame #0 {
                    n153 = while {
                      tunnel: w278 -> [w285]
                      tunnel: w277 -> [w284]
                      tunnel: w276 -> [w283]
                      stop <- w279 stop-if-true
                      n154 = Wait (ms)(milliseconds to wait=u32 5) -> ()  [unwired: 1 out]
                      n155 = call "Motor Ramp.vi"("Command limit"=w283, "Joystick in"=0.8) -> ("Joystick out"=w282:dbl)  [unwired: 9 in]
                      n156 = global read "Robot Global Data.vi" "Loaded?"() -> (w279:bool)
                      n157 = call <vilib>:"WPI_MotorControlSetOutput.vi"("error in (no error)"=w284, "Output"=w282, "MotorControlDevRef"=w285) -> ()  [unwired: 6 in, 3 out]
                    }
                  }
                  frame #1 {
                    n158 = call "Motor Ramp.vi"("Command limit"=w289, "Joystick in"=0.0) -> ("Joystick out"=w288:dbl)  [unwired: 9 in]
                    n159 = call <vilib>:"WPI_MotorControlSetOutput.vi"("error in (no error)"=w290, "Output"=w288, "MotorControlDevRef"=w286) -> ()  [unwired: 6 in, 3 out]
                  }
                }
              }
            }
          }
        }
        n160 = Wait (ms)(milliseconds to wait=u32 5) -> ()  [unwired: 1 out]
      }
    }
    frame Disabled {
    }
  }
  n161 = disable-structure shown="Enabled" {
    frame Enabled {
      n162 = call <vilib>:"WPI_PotentiometerRefNum Registry Get.vi"("refnum name"="Pot") -> ("PotDevRef"=w293:T9)  [unwired: 9 in, 1 out]
      n163 = call-poly <vilib>:"WPI_UltrasonicRefNum Registry Get.vi"("refnum name"="Sonar") -> ("SonarMB1010DigitalDevRef"=w292:T13)  [unwired: 9 in, 1 out]
      n164 = call "Z900_navX_RefNum_Get.vi"("refnum name"="NavX") -> ("navX Device"=w295:T16)  [unwired: 9 in, 1 out]
      n165 = while {
        tunnel: w295 -> [w307]
        tunnel: w293 -> [w303]
        tunnel: w292 -> [w301]
        stop <- FALSE stop-if-true
        # "NavX Status"
        n166 = call "Z900_navX_Get_YPRHfH.vi"("navX Device"=w307) -> ("YRPHfH"=w304:T18, "navX Device"=w306:T16)  [unwired: 7 in, 2 out]
        n167 = Wait (ms)(milliseconds to wait=u32 10) -> ()  [unwired: 1 out]
        n168 = Unbundle By Name(w304) -> ("Pitch"=→"Pitch":dbl, "Roll"=→"Roll":dbl, "Yaw"=→"Yaw":dbl)
        n169 = case shown="True" "Yaw Reset" {
          tunnel: w306 -> [_ w312]
          frame False {
          }
          frame True {
            n170 = call "Z900_navX_Set_ZeroYaw.vi"("navX Device"=w312) -> ()  [unwired: 9 in, 2 out]
          }
        }
        n171 = call <vilib>:"WPI_Power Get PDP Currents.vi"("PDP Channel"=10) -> ("current (A)"=→"current (A)":dbl)  [unwired: 12 in, 2 out]
        n172 = call-poly <vilib>:"WPI_UltrasonicGetRange.vi"("SonarMB1010DigitalDevRef"=w301) -> ("Distance"=→"Distance":dbl)  [unwired: 8 in, 2 out]
        n173 = call <vilib>:"WPI_PotentiometerGetNormalized.vi"("PotDevRef"=w303) -> ("Normalized Value"=→"Potentiometer":dbl)  [unwired: 8 in, 2 out]
      }
    }
    frame Disabled {
    }
  }
  n174 = disable-structure shown="Enabled" {
    frame Enabled {
      # "Intakearm OVERRIDE"
      n175 = call <vilib>:"WPI_MotorControlRefNum Registry Get.vi"("refnum name"="Arm 1") -> ("MotorControlDevRef"=w314:T2)  [unwired: 9 in, 1 out]
      n176 = call <vilib>:"WPI_MotorControlRefNum Registry Get.vi"("refnum name"="Arm 2") -> ("MotorControlDevRef"=w313:T2)  [unwired: 9 in, 1 out]
      n177 = while {
        tunnel: w314 -> [w319]
        tunnel: w313 -> [w318]
        stop <- FALSE stop-if-true
        n178 = global read "Robot Global Data.vi" "btn_intake_override"() -> (w317:bool)
        n179 = Wait (ms)(milliseconds to wait=u32 10) -> ()  [unwired: 1 out]
        n180 = case shown="True" w317 {
          tunnel: w319 -> [_ w330]
          tunnel: w318 -> [_ w329]
          frame False {
          }
          frame True {
            w325 = 0.35 ("t")
            n181 = global read "Robot Global Data.vi" "btn_intakearm_down (manual)"() -> (w326:bool)
            n182 = global read "Robot Global Data.vi" "btn_intakearm_up (manual)"() -> (w323:bool)
            n183 = Negate(x=w325) -> (-x=w324:dbl)
            n184 = Select(t=w325, s=w326, f=0.0) -> (s? t:f=w328:dbl)
            n185 = Select(t=w324, s=w323, f=w328) -> (s? t:f=w322:dbl)
            n186 = call <vilib>:"WPI_MotorControlSetOutput.vi"("Output"=w322, "MotorControlDevRef"=w330) -> ()  [unwired: 7 in, 3 out]
            n187 = call <vilib>:"WPI_MotorControlSetOutput.vi"("Output"=w322, "MotorControlDevRef"=w329) -> ()  [unwired: 7 in, 3 out]
          }
        }
      }
    }
    frame Disabled {
    }
  }
  n188 = disable-structure shown="Enabled" {
    frame Enabled {
      # "Scaler OVERRIDE"
      n189 = call <vilib>:"WPI_MotorControlRefNum Registry Get.vi"("refnum name"="Scaler Lift 2") -> ("MotorControlDevRef"=w333:T2)  [unwired: 9 in, 1 out]
      n190 = call <vilib>:"WPI_MotorControlRefNum Registry Get.vi"("refnum name"="Scaler Lift 1") -> ("MotorControlDevRef"=w331:T2)  [unwired: 9 in, 1 out]
      n191 = call <vilib>:"WPI_MotorControlRefNum Registry Get.vi"("refnum name"="Scaler") -> ("MotorControlDevRef"=w334:T2)  [unwired: 9 in, 1 out]
      n192 = while {
        tunnel: w334 -> [w340]
        tunnel: w333 -> [w339]
        tunnel: w331 -> [w337]
        stop <- FALSE stop-if-true
        n193 = global read "Robot Global Data.vi" "btn_scaler_override"() -> (w338:bool)
        n194 = Wait (ms)(milliseconds to wait=u32 10) -> ()  [unwired: 1 out]
        n195 = case shown="True" w338 {
          tunnel: w340 -> [_ w350]
          tunnel: w339 -> [_ w349]
          tunnel: w337 -> [_ w348]
          frame False {
          }
          frame True {
            n196 = global read "Robot Global Data.vi" "axis_lift(manual)"() -> (w344:dbl)
            n197 = global read "Robot Global Data.vi" "axis_scaler (manual)"() -> (w347:dbl)
            n198 = Negate(x=w344) -> (-x=w343:dbl)
            n199 = call <vilib>:"WPI_MotorControlSetOutput.vi"("Output"=w343, "MotorControlDevRef"=w349) -> ()  [unwired: 7 in, 3 out]
            n200 = call <vilib>:"WPI_MotorControlSetOutput.vi"("Output"=w343, "MotorControlDevRef"=w348) -> ()  [unwired: 7 in, 3 out]
            n201 = Multiply(x=w347, y=0.5) -> (x*y=w346:dbl)
            n202 = call <vilib>:"WPI_MotorControlSetOutput.vi"("Output"=w346, "MotorControlDevRef"=w350) -> ()  [unwired: 7 in, 3 out]
          }
        }
      }
    }
    frame Disabled {
    }
  }
